vi "FPGA_controller.vi"() -> ()   [LabVIEW 2017]
uses:
  <vilib>/rvi/Emulation/niFpgaGetClockAttributes.vi
  <vilib>/rvi/Emulation/niFpgaSctlEmulationGetInTimedLoop.vi
  <vilib>/rvi/Emulation/niFpgaEmulationReportErrorSimple.vi
  <vilib>/rvi/eio/common/nirviEmuTemplateMethod_errors.vi
  <vilib>/rvi/Emulation/niFpgaCriticalErrorInLSC.vi
  <vilib>/eio/EIONode/EIONode.xnode
panel:
  out "VALID":bool
  in  "Scale x2":fxp<+/-,32,16>=10.0 format="%#_21g"
  in  "m_first x2":fxp<+/-,49,33>=4.9499969482421875 format="%#_26g"
  in  "Offset x2":fxp<+/-,48,32> format="%#_26g"
  in  "1/eta x":fxp<+/-,32,16>=200.0 format="%#_21g"
  in  "m_first x1":fxp<+/-,49,33>=0.649993896484375 format="%#_26g"
  in  "Offset x1":fxp<+/-,48,32> format="%#_26g"
  in  "Scale x1":fxp<+/-,32,16>=5.0 format="%#_21g"
  in  "stop 2":bool
  # "STATES CONVERSION"
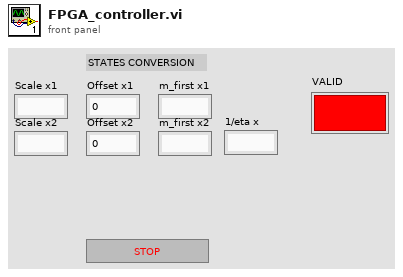
[diagram p1: front panel]
types:
  T1 = cluster{"Boolean array[0]":bool, "Boolean array[1]":bool, "Boolean array[2]":bool, "Boolean array[3]":bool, "Boolean array[4]":bool, "Boolean array[5]":bool, "Boolean array[6]":bool, "Boolean array[7]":bool, "Boolean array[8]":bool, "Boolean array[9]":bool, "Boolean array[10]":bool, "Boolean array[11]":bool, "Boolean array[12]":bool, "Boolean array[13]":bool, "Boolean array[14]":bool, "Boolean array[15]":bool}
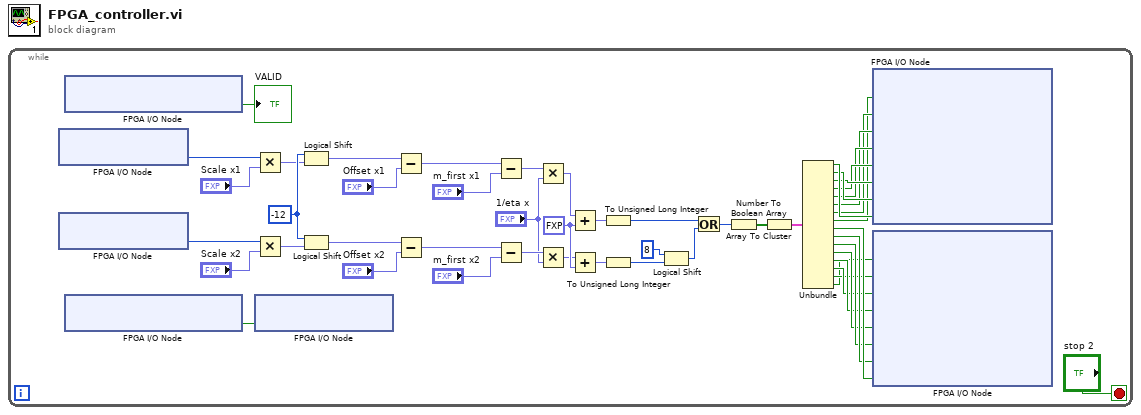
[diagram p0: block diagram]
diagram:
  n1 = while {
    stop <- "stop 2" stop-if-true
    w25 = fxp<+/-,64,32> 0.5 ("y")
    w23 = i16 -12 ("y")
    n2 = xnode "FPGA I/O Node"() -> ("ConnectorA/AI0"=w9:u16)  [unwired: 1 in, 1 out]
    n3 = xnode "FPGA I/O Node"() -> ("ConnectorA/AI1"=w7:u16)  [unwired: 1 in, 1 out]
    n4 = xnode "FPGA I/O Node"() -> ("Component-Level IP\\po1"=→"VALID":bool)  [unwired: 1 in, 1 out]
    n5 = xnode "FPGA I/O Node"() -> ("Component-Level IP\\po0"=w32:bool)  [unwired: 1 in, 1 out]
    n6 = Multiply(x=w9, y="Scale x1") -> (x*y=w22:fxp<+/-,48,32>)
    n7 = Multiply(x=w7, y="Scale x2") -> (x*y=w26:fxp<+/-,48,32>)
    n8 = xnode "FPGA I/O Node"("ConnectorA/DIO0"=w32) -> ()  [unwired: 1 in, 1 out]
    n9 = Logical Shift(y=w23, x=w22) -> (x << y=w19:fxp<+/-,48,32>)
    n10 = Logical Shift(y=w23, x=w26) -> (x << y=w16:fxp<+/-,48,32>)
    n11 = Subtract(x=w19, y="Offset x1") -> (x-y=w20:fxp<+/-,49,33>)
    n12 = Subtract(x=w16, y="Offset x2") -> (x-y=w17:fxp<+/-,49,33>)
    n13 = Subtract(x=w20, y="m_first x1") -> (x-y=w21:fxp<+/-,50,34>)
    n14 = Subtract(x=w17, y="m_first x2") -> (x-y=w15:fxp<+/-,50,34>)
    n15 = Multiply(x=w21, y="1/eta x") -> (x*y=w18:fxp<+/-,64,49>)
    n16 = Multiply(x=w15, y="1/eta x") -> (x*y=w14:fxp<+/-,64,49>)
    n17 = Add(x=w18, y=w25) -> (x+y=w31:fxp<+/-,64,50>)
    n18 = Add(x=w14, y=w25) -> (x+y=w24:fxp<+/-,64,50>)
    n19 = To Unsigned Long Integer(number=w31) -> (unsigned 32bit integer=w27:u32)
    n20 = To Unsigned Long Integer(number=w24) -> (unsigned 32bit integer=w29:u32)
    n21 = Logical Shift(y=8, x=w29) -> (x << y=w28:u32)
    n22 = Or(x=w27, y=w28) -> (x .or. y?=w10:u32)
    n23 = Number To Boolean Array(number=w10) -> (Boolean array=w11:bool[])
    n24 = Array To Cluster(array=w11) -> (cluster=w49:T1)
    n25 = Unbundle(w49) -> ("Boolean array[0]"=w48:bool, "Boolean array[1]"=w47:bool, "Boolean array[2]"=w46:bool, "Boolean array[3]"=w45:bool, "Boolean array[4]"=w44:bool, "Boolean array[5]"=w43:bool, "Boolean array[6]"=w42:bool, "Boolean array[7]"=w41:bool, "Boolean array[8]"=w40:bool, "Boolean array[9]"=w39:bool, "Boolean array[10]"=w38:bool, "Boolean array[11]"=w37:bool, "Boolean array[12]"=w36:bool, "Boolean array[13]"=w35:bool, "Boolean array[14]"=w34:bool, "Boolean array[15]"=w33:bool)
    n26 = xnode "FPGA I/O Node"("Component-Level IP\\pi00"=w41, "Component-Level IP\\pi01"=w42, "Component-Level IP\\pi02"=w43, "Component-Level IP\\pi03"=w44, "Component-Level IP\\pi04"=w45, "Component-Level IP\\pi05"=w46, "Component-Level IP\\pi06"=w47, "Component-Level IP\\pi07"=w48) -> ()  [unwired: 8 in, 8 out]
    n27 = xnode "FPGA I/O Node"("Component-Level IP\\pi08"=w33, "Component-Level IP\\pi09"=w34, "Component-Level IP\\pi10"=w35, "Component-Level IP\\pi11"=w36, "Component-Level IP\\pi12"=w37, "Component-Level IP\\pi13"=w38, "Component-Level IP\\pi14"=w39, "Component-Level IP\\pi15"=w40) -> ()  [unwired: 8 in, 8 out]
  }
